vi "SeperateTest.vi"() -> ()   [LabVIEW 2019]
uses:
  <vilib>/myRIO/Common/Instrument Driver Framework/myRIO v1.0/Encoder/typedefs/Encoder Signal Mode.ctl
  <vilib>/myRIO/Instrument Drivers/Onboard IO/Encoder/typedefs/Encoder Reference.ctl
  <vilib>/myRIO/Common/Instrument Driver Framework/Utilities/typedefs/myRIO Generic Hardware Reference.ctl
  <vilib>/myRIO/Common/Instrument Driver Framework/Utilities/typedefs/Hardware Version Enum.ctl
  <vilib>/myRIO/Common/Instrument Driver Framework/Utilities/typedefs/myRIO v1.0 Reference.ctl
  <vilib>/myRIO/Common/Instrument Driver Framework/Utilities/typedefs/Generic FPGA Reference.ctl
  <vilib>/myRIO/Common/Instrument Driver Framework/myRIO v1.0/Encoder/typedefs/Encoder Channels Enum.ctl
  <vilib>/myRIO/Common/Instrument Driver Framework/myRIO v1.0/Encoder/typedefs/Encoder Configuration v1.0.ctl
  <vilib>/userDefined/High Color/nirio_resource_hc.ctl
  <vilib>/myRIO/Common/Instrument Driver Framework/Utilities/vis/Is FPGA Ref Available.vi
  <vilib>/myRIO/Common/Instrument Driver Framework/myRIO v1.0/Encoder/vis/myRIO v1.1 Open Encoder.vi
  <vilib>/myRIO/Instrument Drivers/Onboard IO/Encoder/vis/Read.vi
  <vilib>/myRIO/Common/Instrument Driver Framework/Utilities/vis/Validate Channels.vi
  <vilib>/myRIO/Common/Instrument Driver Framework/myRIO v1.0/Encoder/vis/myRIO v1.0 Reserve Encoder.vi
  <vilib>/myRIO/Common/Instrument Driver Framework/myRIO v1.0/UART/vis/myRIO v1.0 Close UART.vi
  <vilib>/myRIO/Common/Instrument Driver Framework/myRIO v1.0/Encoder/vis/myRIO v1.0 Build MUX Configuration Encoder.vi
  <vilib>/myRIO/Common/Instrument Driver Framework/myRIO v1.0/Resource Manager/vis/myRIO v1.0 Reserve Channel List.vi
  <vilib>/myRIO/Common/Instrument Driver Framework/myRIO v1.0/Resource Manager/vis/myRIO v1.0 Create Configuration List.vi
  <vilib>/myRIO/Common/Instrument Driver Framework/myRIO v1.0/Resource Manager/vis/myRIO v1.0 Reserve Channel.vi
  <vilib>/myRIO/Common/Instrument Driver Framework/myRIO v1.0/Resource Manager/vis/myRIO v1.0 Unreserve Channel.vi
  <vilib>/myRIO/Common/Instrument Driver Framework/myRIO v1.0/Resource Manager/vis/myRIO v1.0 Build Mutex Name.vi
  <vilib>/Utility/VariantDataType/GetNumericInfo.vi
  <vilib>/Utility/error.llb/Error Cluster From Error Code.vi
  <vilib>/myRIO/Common/Instrument Driver Framework/myRIO v1.0/myRIO v1.1 Open.vi
  <vilib>/myRIO/Common/Instrument Driver Framework/Utilities/vis/IO Manager.vi
  <vilib>/myRIO/Common/Instrument Driver Framework/Utilities/vis/Configuration Manager.vi
  <vilib>/myRIO/Common/Instrument Driver Framework/myRIO v1.0/Resource Manager/vis/myRIO v1.0 Configure IO.vi
  <vilib>/myRIO/Common/Instrument Driver Framework/myRIO v1.0/myRIO v1.0 Close.vi
  <vilib>/myRIO/Common/Instrument Driver Framework/myRIO v1.0/Encoder/vis/myRIO v1.0 Configure Encoder.vi
  <vilib>/myRIO/Common/Instrument Driver Framework/myRIO v1.0/Encoder/vis/myRIO v1.0 Read Encoder.vi
  <vilib>/Utility/file.llb/Write Delimited Spreadsheet (DBL).vi
  <vilib>/myRIO/Common/Instrument Driver Framework/Utilities/vis/FPGA Ref Manager.vi
  <vilib>/myRIO/Common/Instrument Driver Framework/myRIO v1.0/myRIO v1.0 Reset FPGA.vi
  <vilib>/myRIO/Common/Instrument Driver Framework/myRIO v1.0/IRQ/vis/myRIO v1.0 IRQ Info FGV.vi
  <vilib>/myRIO/Common/Instrument Driver Framework/myRIO v1.0/IRQ/vis/myRIO v1.0 Timer IRQ Info FGV.vi
  <vilib>/myRIO/Common/Instrument Driver Framework/myRIO v1.0/IRQ/vis/myRIO v1.0 ISR Agent.vi
  <vilib>/myRIO/Instrument Drivers/Utilities/vis/Reset Index.vi
  <vilib>/myRIO/Common/Instrument Driver Framework/myRIO v1.0/Resource Manager/vis/myRIO v1.0 Block Write Resource Manager.vi
  <vilib>/myRIO/Express VI/Onboard IO/Encoder/Encoder Express VI.xnode
  <vilib>/myRIO/Common/Instrument Driver Framework/myRIO v1.0/Encoder/typedefs/Encoder Count Direction Enum.ctl
  <vilib>/myRIO/Instrument Drivers/Onboard IO/Encoder/vis/myRIO Encoder Open.xnode
  <vilib>/myRIO/Instrument Drivers/Onboard IO/Encoder/Encoder.lvlib
  <vilib>/myRIO/Instrument Drivers/Utilities/Utilities.lvlib
panel:
  in  "ref pos 2":dbl
  in  "ref pos 1":dbl
  out "error out":errorcluster
  in  "Stop 2":bool
  out "Direction 1":enum16{"Counting Up", "Counting Down"}(ring)
  out "Overflow? 1":bool
  in  "Reset":bool
  out "Graph 3":cluster{"ref 1":dbl, "rads":dbl}(graph)
  in  "Freq[Hz]":dbl=1000.0
  out "Direction 2":enum16{"Counting Up", "Counting Down"}(ring)
  out "Overflow? 2":bool
  in  "Reset 2":bool
  out "ref pos 1":dbl
  out "Duty Cycle out 2":dbl=0.5
  out "Duty Cycle out":dbl=0.5
  out "Graph 2":cluster{dbl, "x2hat":dbl}(graph)
  out "ref pos 2":dbl
  out "pos 1":dbl
  out "pos2":dbl
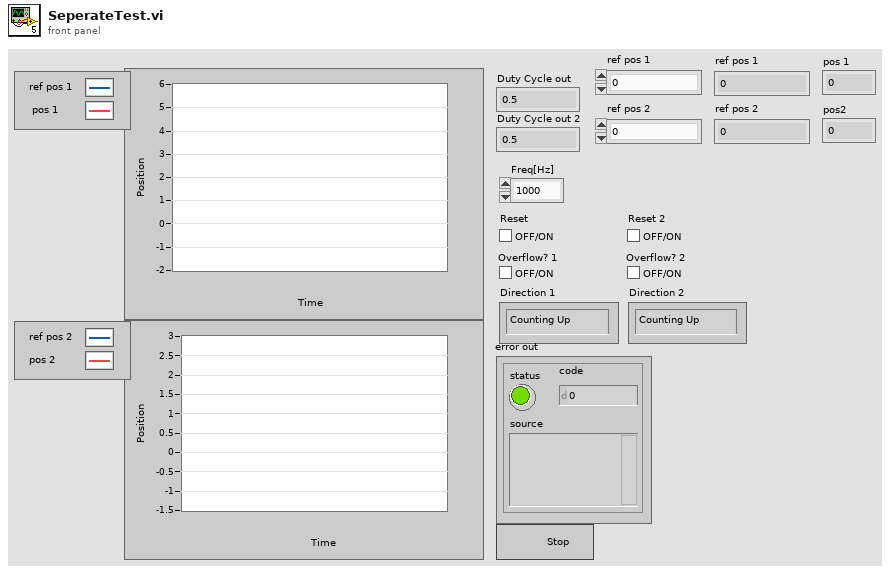
[diagram p1: front panel]
types:
  T1 = typedef "Encoder.lvlib/Encoder Reference.ctl" = cluster{"myRIO Reference":T2, "Encoder Channels Enum":T6}
  T2 = typedef "myRIO Generic Hardware Reference.ctl" = cluster{"myRIO Model":T3, "myRIO Hardware Reference":T4}
  T3 = typedef "Hardware Version Enum.ctl" = enum16{"Unknown", "myRIO-1900", "myRIO-1950", "roboRIO", "NI ELVIS RIO CM", "ELVIS III"}
  T4 = typedef "myRIO v1.0 Reference.ctl" = cluster{"Generic FPGA Reference":T5, "Allow multiple opens":bool}
  T5 = typedef "Generic FPGA Reference.ctl" = refnum<k20>
  T6 = typedef "Encoder Channels Enum.ctl" = enum16{"Not Connected", "C/ENC0", "C/ENC1", "A/ENC", "A/ENC0", "A/ENC1", "A/ENC2", "A/ENC3", "A/ENC4", "A/ENC5", "A/ENC6", "A/ENC7", "A/ENC8", "A/ENC9", "B/ENC", "B/ENC0", "B/ENC1", "B/ENC2", "B/ENC3", "B/ENC4", "B/ENC5", "B/ENC6", "B/ENC7", "B/ENC8", "B/ENC9", "DIO/ENC0", "DIO/ENC1", "DIO/ENC2", "DIO/ENC3", "DIO/ENC4"}
  T7 = typedef "Encoder Signal Mode.ctl" = enum16{"Quadrature phase signal", "Step and direction signal"}
  T8 = typedef "nirio_resource_hc.ctl" = tag
  T9 = typedef "Encoder Count Direction Enum.ctl" = enum16{"Counting Up", "Counting Down"}
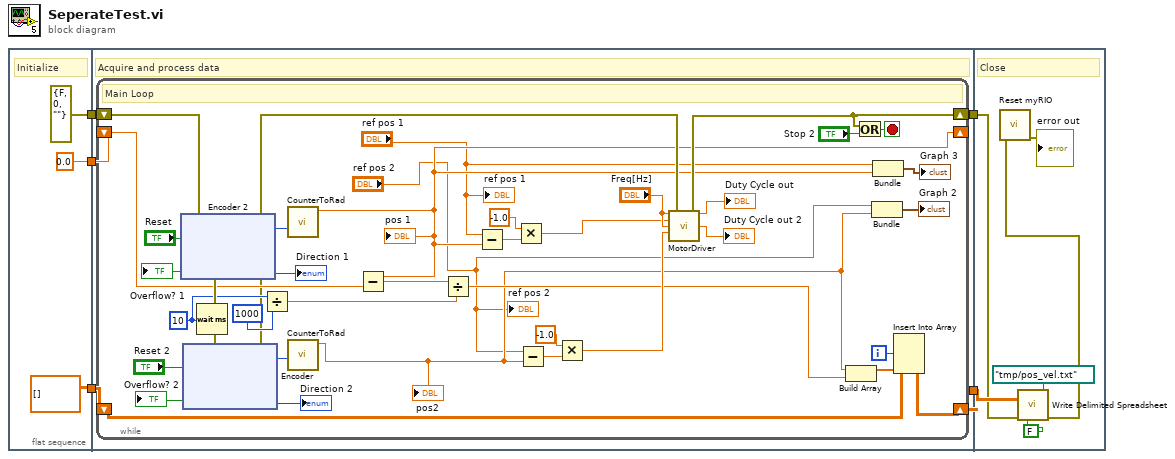
[diagram p0: block diagram]
diagram:
  n1 = flat-sequence {
    tunnel: [errorcluster {"status"=FALSE, "code"=0, "source"=""} ("error in (no error)")] -> w5
    tunnel: [dbl[][] [] ("array")] -> w4
    tunnel: [0.0 ("rads")] -> w3
    tunnel: w5 -> [w13]
    tunnel: w4 -> [w12]
    tunnel: [w11] -> w2
    tunnel: [w10] -> w1
    tunnel: w3 -> [w9]
    tunnel: w2 -> [w148]
    tunnel: w1 -> [w149]
    frame #0 {
      # "Initialize"
    }
    frame #1 {
      # "Acquire and process data"
      n2 = while {
        shift-right: [w21] -> w11
        shift-left: w13 -> [w44]
        shift-right: [w47] -> w10
        shift-left: w12 -> [w46]
        shift-right: [w16] -> _
        shift-left: w9 -> [w34]
        i -> [w43]
        stop <- w51 stop-if-true
        w35 = u32 10 ("milliseconds to wait")
        # "Main Loop"
        n3 = xnode "Encoder 2"("error in (no error)"=w44, "Reset Counter"="Reset") -> ("error out"=w39:errorcluster, "Counter Value"=w33:i32, "Counter Direction"=→"Direction 1":T9, "Overflow?"=→"Overflow? 1":bool)
        n4 = xnode "Encoder"("error in (no error)"=w39, "Reset Counter"="Reset 2") -> ("error out"=w22:errorcluster, "Counter Value"=w32:i32, "Counter Direction"=→"Direction 2":T9, "Overflow?"=→"Overflow? 2":bool)
        n5 = Wait (ms)(milliseconds to wait=w35) -> ()  [unwired: 1 out]
        n6 = Divide(x=w35, y=u32 1000) -> (x/y=w38:dbl)
        n7 = call "CounterToRad.vi"("Counter Value"=w33) -> ("rads"=w16:dbl)  [unwired: 10 in]
        "pos 1" <- w16
        n8 = call "CounterToRad.vi"("Counter Value"=w32) -> ("rads"=w19:dbl)  [unwired: 10 in]
        "pos2" <- w19
        n9 = Subtract(x=w16, y=w34) -> (x-y=w37:dbl)
        n10 = Divide(x=w37, y=w38) -> (x/y=w20:dbl)
        n11 = Subtract(x="ref pos 1", y=w16) -> (x-y=w28:dbl)
        n12 = Multiply(x=-1.0 ("vel ref"), y=w28) -> (x*y=w26:dbl)
        n13 = Subtract(x="ref pos 2", y=w19) -> (x-y=w25:dbl)
        n14 = Multiply(x=-1.0 ("vel ref"), y=w25) -> (x*y=w23:dbl)
        n15 = call "MotorDriver.vi"("Frequency [Hz]"="Freq[Hz]", "Duty Cycle in"=w26, "Frequency [Hz] 2"="Freq[Hz]", "Duty Cycle in 2"=w23, "error in (no error)"=w22) -> ("Duty Cycle out"=→"Duty Cycle out":dbl, "Duty Cycle out 2"=→"Duty Cycle out 2":dbl, "error out"=w21:errorcluster)  [unwired: 8 in]
        n16 = Build Array(w19, w20) -> (w45:dbl[])
        n17 = Or(x=w21, y="Stop 2") -> (x .or. y?=w51:bool)
        n18 = Bundle("ref pos 2"="ref pos 2", "rads"=w19) -> (→"Graph 2":cluster{"ref pos 2":dbl, "rads":dbl})  [unwired: 1 in]
        n19 = Bundle("ref pos 1"="ref pos 1", "rads"=w16) -> (→"Graph 3":cluster{"ref pos 1":dbl, "rads":dbl})  [unwired: 1 in]
        n20 = Insert Into Array(array=w46, index (row)=w43, new element=w45) -> (w47:dbl[][])  [unwired: 1 in]
        "ref pos 1" <- "ref pos 1"
        "ref pos 2" <- "ref pos 2"
      }
    }
    frame #2 {
      # "Close"
      n21 = call-poly <vilib>:"Write Delimited Spreadsheet.vi"("file path (dialog if empty)"=path "/tmp/pos_vel.txt", "2D data"=w149, "error in (no error)"=w148, "transpose? (no:F)"=FALSE) -> ("error out"=w147:errorcluster)  [unwired: 10 in, 1 out]
      n22 = call <vilib>:"Reset myRIO.vi"("error in (no error)"=w147) -> ("error out"=→"error out":errorcluster)  [unwired: 10 in]
    }
  }
